vi "Basic Operations (numeric).vi"(8 "Operation":T1, 10 "x":dbl, 11 "y":dbl) -> (3 "x op y":dbl)   [LabVIEW 2024, in "Libreria de reuso.lvlib"]
uses:
  Libreria de reuso.lvlib
  Operation--enum.ctl
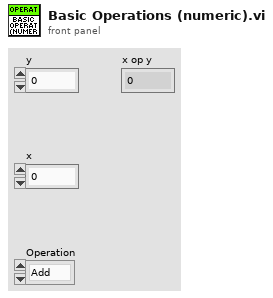
[diagram p1: front panel]
types:
  T1 = typedef "Libreria de reuso.lvlib/Operation--enum.ctl" = enum16{"Add", "Subtract", "Multiply", "Divide"}
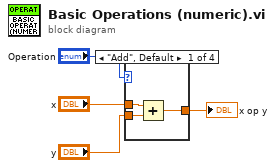
[diagram p0: block diagram]
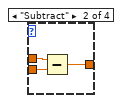
[diagram p2: hidden frame]
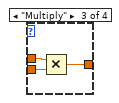
[diagram p3: hidden frame]
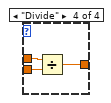
[diagram p4: hidden frame]
diagram:
  n1 = case shown="\"Add\", Default" "Operation" {
    tunnel: "y" -> [w7 w10 w13 w16]
    tunnel: "x" -> [w6 w9 w12 w15]
    tunnel: [w5 w8 w11 w14] -> w2
    frame "Add", Default {
      n2 = Add(x=w6, y=w7) -> (x+y=w5:dbl)
    }
    frame "Subtract" {
      n3 = Subtract(x=w9, y=w10) -> (x-y=w8:dbl)
    }
    frame "Multiply" {
      n4 = Multiply(x=w12, y=w13) -> (x*y=w11:dbl)
    }
    frame "Divide" {
      n5 = Divide(x=w15, y=w16) -> (x/y=w14:dbl)
    }
  }
  "x op y" <- w2
